vi "Translation_GetDistance.vi"(9 "other Translation":T1, 11 "In Translation":T1) -> (2 "Distance":dbl)   [LabVIEW 2019, in "Trajectory_Library.lvlib"]
doc: "Calculates the distance between two translations in 2d space.\n\nThis function uses the pythagorean theorem to calculate the distance. distance = sqrt((x2 - x1)^2 + (y2 - y1)^2)\n\nParameters: \n - IN TRANSLATION - This TRANSLATION data structure\n - OTHER TRANSLATION - The translation to compute the distance to.\n\nReturns:\n - Distance - The distance between the two translations."
uses:
  Trajectory_Library.lvlib
  TRANSLATION2D.ctl
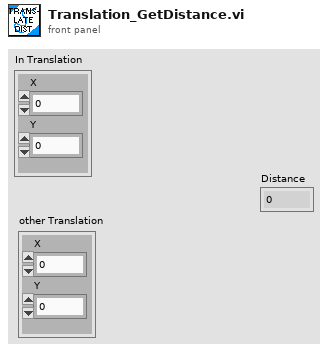
[diagram p1: front panel]
types:
  T1 = typedef "Trajectory_Library.lvlib/TRANSLATION2D.ctl" = cluster{"X":dbl, "Y":dbl}
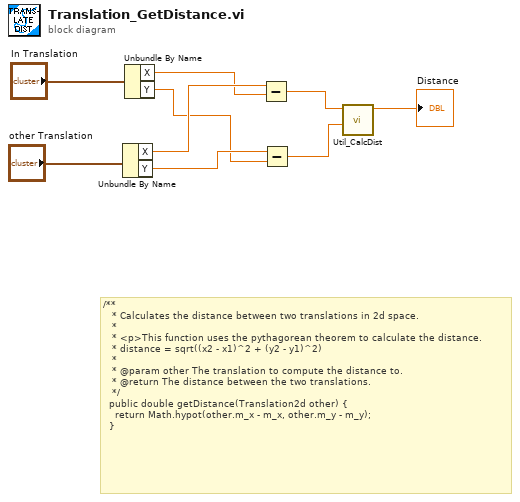
[diagram p0: block diagram]
diagram:
  # "/**\n   * Calculates the distance between two translations in 2d space.\n   *\n   * <p>This function uses the pythagorean theorem to calculate the distance.\n   * distance = sqrt((x2 - x1)^2 + (y2 - y1)^2)\n   *\n   * @param other The translation to compute the distance to.\n   * @return The distance between the two translations.\n   */\n  public double getDistance(Translation2d other) {\n    return Math.hypot(other.m_x - m_x, other.m_y - m_y);\n  }"
  n1 = Unbundle By Name("other Translation") -> ("X"=w7:dbl, "Y"=w5:dbl)
  n2 = Unbundle By Name("In Translation") -> ("X"=w6:dbl, "Y"=w4:dbl)
  n3 = Subtract(x=w7, y=w6) -> (x-y=w3:dbl)
  n4 = Subtract(x=w5, y=w4) -> (x-y=w2:dbl)
  n5 = call "Util_CalcDist.vi"("Y"=w2, "X"=w3) -> ("DIST"=→"Distance":dbl)  [unwired: 9 in]
